vi "MrClean.init clean afg.vi"(0 "i ref in":refnum<vi>, 1 "CleanAfg":i32, 2 "amplitude [V]":dbl format="%.2f", 3 "ms timeout (100)":i32=100, 4 "frequency [Hz]":dbl format="%.2f", 5 "error in (no error)":errorcluster) -> (14 "i ref out":refnum<vi>, 17 "timed out":bool, 19 "error out":errorcluster)   [LabVIEW 2014, in "MrClean.lvlib"]
doc: "Sets the frequency [Hz] and amplitude [V] at the AFG with number CleanAFG. The numbering of the CleanAFGs starts with 0."
uses:
  MrClean.lvlib
  CS_Core/CSSystem/CoreDefs/CoreDefs.error_type.ctl
  CS_Core/CSSystem/CoreLib/CoreLib.double 2 byte array.vi
  CS_Core/CSSystem/CoreLib/CoreLib.lvlib
  CS_Core/BaseProcess/BaseProcess.lvlib
  LEBITLib/LEBITLib.lvlib
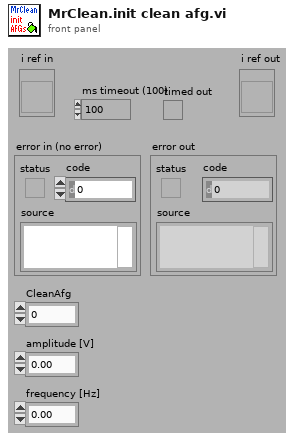
[diagram p1: front panel]
types:
  T1 = typedef "CoreDefs.error_type.ctl" = enum16{"no error", "can't load process", "can't unload process", "process does not exist", "can't install process", "can't remove process", "unknown function", "time out", "can't execute function", "duplicate queue name", "super not found", "caller queue invalid", "can't ping process", "unknown error", "VISA Error", "VISA timeout", "GPIB timeout", "GPIB error", "communication error", "data type mismatch", "can't read data from OPC server", "can't write data to OPC server", "OET error", "function not implemented", "process already exists", "invalid Shared Variable name", "error writing Shared Variable", "error reading Shared Variable", "invalid client name", "corrupt database", "unknown class", "call not authorized", "parameter out of range", "OET timeout: can't get data to modify", "invalid queue name", "requested operation incompatible with current state", "event undefined", "event disabled", "state undefined", "caller is not a friend", "EventBuilder: bad eventID", "EventBuilder: no DAQ devices", "a thread must not stop itself", "UNUSED ELEMENT4", "DiscArchiver: eventData incomplete", "DiscArchiver: eventData does not belong to run", "DiscArchiver: can't open file", "DiscArchiver: can't write to file", "DiscArchiver: available disc space low", "can't acquire semaphore", "error reading data from database", "notifier object is not existing", "can't register process", "can't unregister process", "illegal event type", "object disabled", "object already exists", "can't change state", "Instrument not found", "no connection to remote node", "invalid reference", "N/A", "UNUSED ELEMENT 1", "element not found", "illegal TCP/IP connection detected", "object does not exist", "invalid access ID", "unknown CS system", "invalid privilige", "unsupported data type", "unsupported server type", "IO server already exists", "Shared Variable already exists"}
  T2 = enum16{"simple", "synchronous", "asynchronous", "notification"}
  T3 = typedef "CoreDefs.rawDataType.ctl" = i8[]
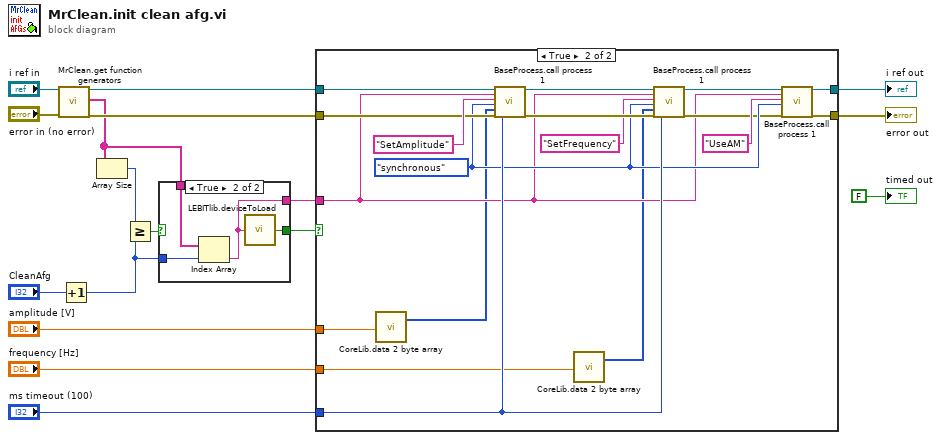
[diagram p0: block diagram]
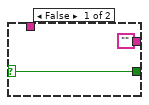
[diagram p2: hidden frame]
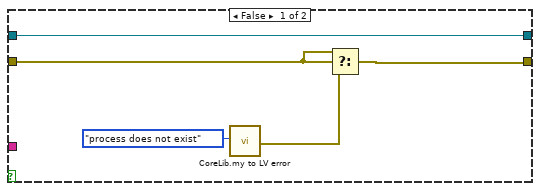
[diagram p3: hidden frame]
diagram:
  n1 = call "MrClean.get function generators.vi"("i ref in"="i ref in", "error in (no error)"="error in (no error)") -> ("i ref out"=w13:refnum<vi>, "function generators"=w3:string[], "error out"=w11:errorcluster)  [unwired: 14 in, 1 out]
  n2 = Increment(x="CleanAfg") -> (x+1=w4:i32)
  n3 = Array Size(array=w3) -> (size(s)=w14:i32)
  n4 = Greater Or Equal?(x=w14, y=w4) -> (x >= y?=w5:bool)
  n5 = case shown="True" w5 {
    selector: w5 -> [w19 _]
    tunnel: ["" w20] -> w1
    tunnel: [w19 w23] -> w2
    tunnel: w4 -> [_ w22]
    tunnel: w3 -> [_ w21]
    frame False {
    }
    frame True {
      n6 = Index Array(array=w21, index=w22) -> (element=w20:string)
      n7 = call "LEBITlib.deviceToLoad.vi"("DeviceName"=w20) -> ("DeviceIsToLoad"=w23:bool)
    }
  }
  n8 = case shown="True" w2 {
    tunnel: [w28 w34] -> w12
    tunnel: w13 -> [w28 w46]
    tunnel: w11 -> [w26 w44]
    tunnel: [w27 w33] -> w10
    tunnel: "amplitude [V]" -> [_ w32]
    tunnel: "frequency [Hz]" -> [_ w30]
    tunnel: "ms timeout (100)" -> [_ w40]
    tunnel: w1 -> [_ w35]
    frame False {
      n9 = call "CoreLib.my to LV error.vi"("ErrorTypes"=CoreDefs.error_type."process does not exist") -> ("myErrorCluster"=w25:errorcluster)  [unwired: 17 in, 1 out]
      n10 = Select(t=w26, s=w26, f=w25) -> (s? t:f=w27:errorcluster)
    }
    frame True {
      w38 = T2."synchronous" ("CallType")
      n11 = call-poly "CoreLib.data 2 byte array.vi"("f64"=w32) -> ("byteArray out"=w31:T3)  [unwired: 18 in]
      n12 = call "BaseProcess.call process 1.vi"("i ref in"=w46, "Object"=w35, "Selector"="SetAmplitude", "CallType"=w38, "Data"=w31, "error in (no error)"=w44, "timeout (ms)"=w40) -> ("i ref out"=w43:refnum<vi>, "error out"=w42:errorcluster)  [unwired: 10 in, 1 out]
      n13 = call-poly "CoreLib.data 2 byte array.vi"("f64"=w30) -> ("byteArray out"=w29:T3)  [unwired: 18 in]
      n14 = call "BaseProcess.call process 1.vi"("i ref in"=w43, "Object"=w35, "Selector"="SetFrequency", "CallType"=w38, "Data"=w29, "error in (no error)"=w42, "timeout (ms)"=w40) -> ("i ref out"=w36:refnum<vi>, "error out"=w37:errorcluster)  [unwired: 10 in, 1 out]
      n15 = call "BaseProcess.call process 1.vi"("i ref in"=w36, "Object"=w35, "Selector"="UseAM", "CallType"=w38, "error in (no error)"=w37) -> ("i ref out"=w34:refnum<vi>, "error out"=w33:errorcluster)  [unwired: 12 in, 1 out]
    }
  }
  "error out" <- w10
  "i ref out" <- w12
  "timed out" <- FALSE ("timed out")
